vi "Ls1 queue ops.vi"(8 "error in (no error)":errorcluster, 11 "Ls1 queue ops":T2(ring)) -> (0 "error out":errorcluster)   [LabVIEW 2017]
uses:
  Type Defs/Ls1 Operations.ctl
panel:
  out "Ls1 Ops 2":T1
  out "Ls1 Ops":T1
  in  "Ls1 Ops":T1
  out "Ls1 queue ops OUT":refnum<queue>
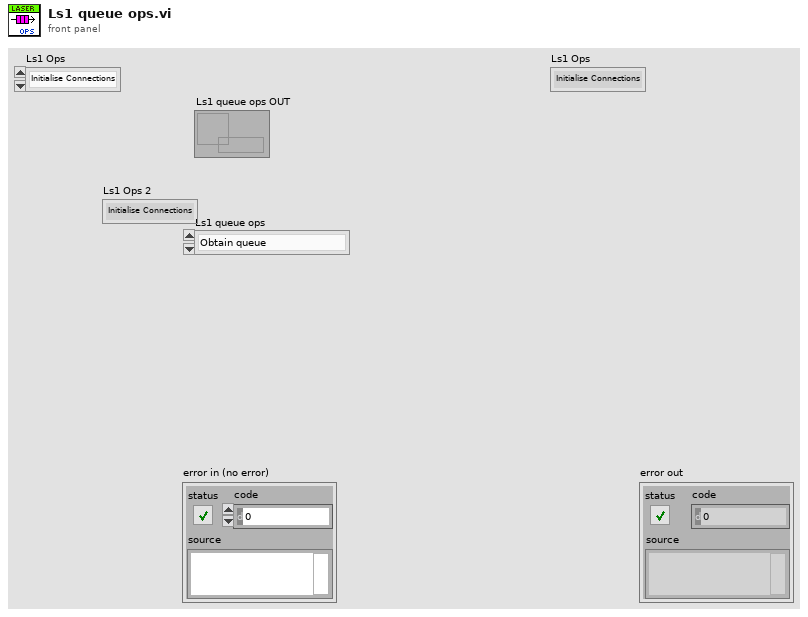
[diagram p1: front panel]
types:
  T1 = typedef "Ls1 Operations.ctl" = enum16{"Initialise Connections", "Initialise system", "Check Status", "Open/Close Shutter", "Start/Stop Pump Peak Hold", "Set wavelength", "Close"}
  T2 = enum16{"Obtain queue", "Enqueue", "Dequeue", "Preview queue", "Get queue status", "Release queue"}
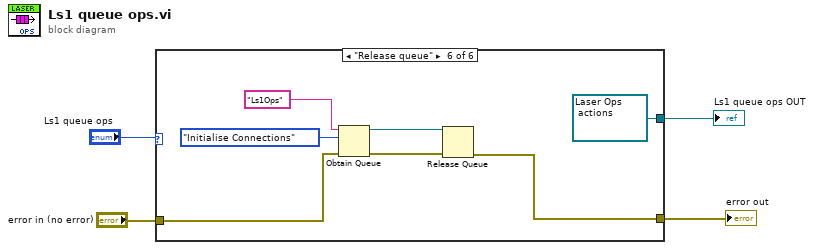
[diagram p0: block diagram]
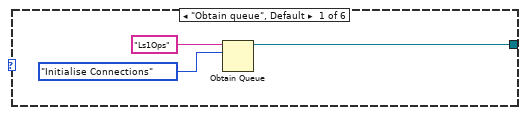
[diagram p2: hidden frame]
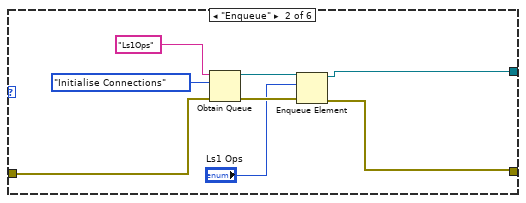
[diagram p3: hidden frame]
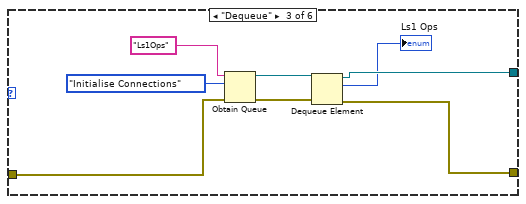
[diagram p4: hidden frame]
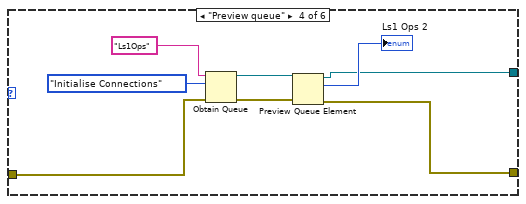
[diagram p5: hidden frame]
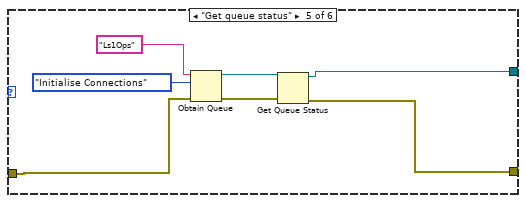
[diagram p6: hidden frame]
diagram:
  n1 = case shown="\"Release queue\"" "Ls1 queue ops" {
    tunnel: [w5 w8 w19 w26 w34 w41] -> w4
    tunnel: "error in (no error)" -> [_ w13 w18 w24 w32 w44]
    tunnel: [_ w11 w17 w25 w33 w40] -> w1
    frame "Obtain queue", Default {
      n2 = Obtain Queue(name (unnamed)="Ls1Ops", element data type=Ls1_Operations."Initialise Connections" ("Laser Ops\n actions")) -> (queue out=w5:refnum<queue>)  [unwired: 3 in, 2 out]
    }
    frame "Enqueue" {
      n3 = Obtain Queue(name (unnamed)="Ls1Ops", element data type=Ls1_Operations."Initialise Connections" ("Laser Ops\n actions"), error in (no error)=w13) -> (queue out=w10:refnum<queue>, error out=w12:errorcluster)  [unwired: 2 in, 1 out]
      n4 = Enqueue Element(queue=w10, element="Ls1 Ops", error in (no error)=w12) -> (queue out=w8:refnum<queue>, error out=w11:errorcluster)  [unwired: 1 in, 1 out]
    }
    frame "Dequeue" {
      n5 = Obtain Queue(name (unnamed)="Ls1Ops", element data type=Ls1_Operations."Initialise Connections" ("Laser Ops\n actions"), error in (no error)=w18) -> (queue out=w20:refnum<queue>, error out=w21:errorcluster)  [unwired: 2 in, 1 out]
      n6 = Dequeue Element(queue=w20, error in (no error)=w21) -> (queue out=w19:refnum<queue>, element=→"Ls1 Ops":T1, error out=w17:errorcluster)  [unwired: 1 in, 1 out]
    }
    frame "Preview queue" {
      n7 = Obtain Queue(name (unnamed)="Ls1Ops", element data type=Ls1_Operations."Initialise Connections" ("Laser Ops\n actions"), error in (no error)=w24) -> (queue out=w28:refnum<queue>, error out=w29:errorcluster)  [unwired: 2 in, 1 out]
      n8 = Preview Queue Element(queue=w28, error in (no error)=w29) -> (queue out=w26:refnum<queue>, element=→"Ls1 Ops 2":T1, error out=w25:errorcluster)  [unwired: 1 in, 1 out]
    }
    frame "Get queue status" {
      n9 = Obtain Queue(name (unnamed)="Ls1Ops", element data type=Ls1_Operations."Initialise Connections" ("Laser Ops\n actions"), error in (no error)=w32) -> (queue out=w36:refnum<queue>, error out=w37:errorcluster)  [unwired: 2 in, 1 out]
      n10 = Get Queue Status(queue=w36, error in (no error)=w37) -> (queue out=w34:refnum<queue>, # pending remove=w35:i32, error out=w33:errorcluster)  [unwired: 1 in, 5 out]
    }
    frame "Release queue" {
      w41 = refnum<queue> refnum items=["Initialise Connections", "Initialise system", "Check Status", "Open/Close Shutter", "Start/Stop Pump Peak Hold", "Set wavelength", "Close"] ("queue out")
      n11 = Obtain Queue(name (unnamed)="Ls1Ops", element data type=Ls1_Operations."Initialise Connections" ("Laser Ops\n actions"), error in (no error)=w44) -> (queue out=w42:refnum<queue>, error out=w43:errorcluster)  [unwired: 2 in, 1 out]
      n12 = Release Queue(queue=w42, error in (no error)=w43) -> (error out=w40:errorcluster)  [unwired: 1 in, 2 out]
    }
  }
  "Ls1 queue ops OUT" <- w4
  "error out" <- w1
